vi "WPI_UtilitiesERRGetRefNum.vi"(8 "error in (no error)":errorcluster) -> (0 "ERRGetRefNum":errorcluster)   [LabVIEW 2017]
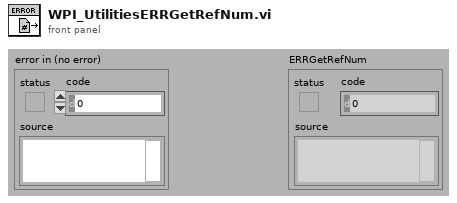
[diagram p1: front panel]
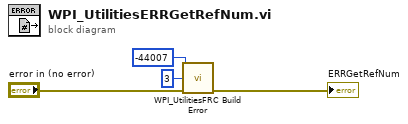
[diagram p0: block diagram]
diagram:
  n1 = call <vilib>:"WPI_UtilitiesFRC Build Error.vi"("error code"=-44007 ("code"), "chain levels to remove (1)"=3, "error in (no error)"="error in (no error)") -> ("error out"=→"ERRGetRefNum":errorcluster)  [unwired: 2 in, 10 out]
